vi "duqugongyi.vi"() -> ()   [LabVIEW 2019]
panel:
  in  "树形控件":string(tree)
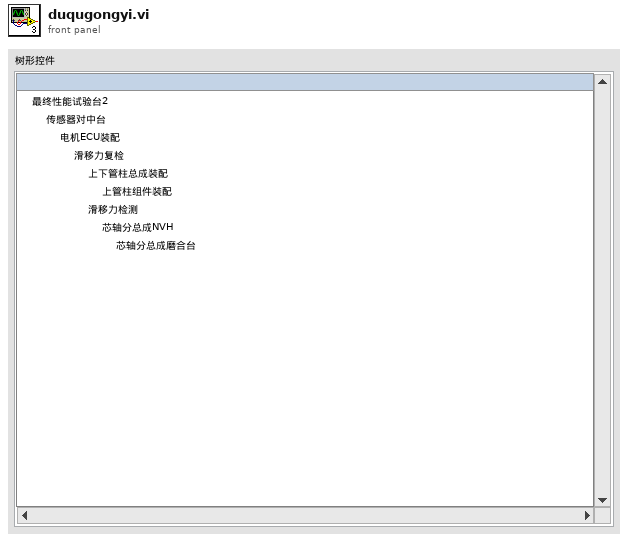
[diagram p1: front panel]
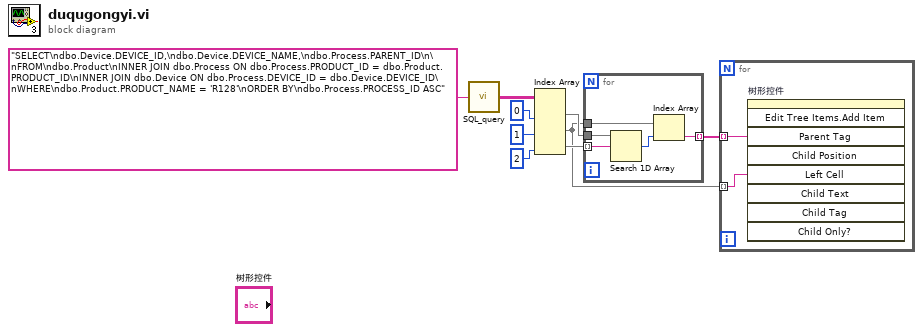
[diagram p0: block diagram]
diagram:
  n1 = call "SQL_query.vi"("SQL query"="SELECT\ndbo.Device.DEVICE_ID,\ndbo.Device.DEVICE_NAME,\ndbo.Process.PARENT_ID\n\nFROM\ndbo.Product\nINNER JOIN dbo.Process ON dbo.Process.PRODUCT_ID = dbo.Product.PRODUCT_ID\nINNER JOIN dbo.Device ON dbo.Process.DEVICE_ID = dbo.Device.DEVICE_ID\nWHERE\ndbo.Product.PRODUCT_NAME = 'R128'\nORDER BY\ndbo.Process.PROCESS_ID ASC") -> ("data"=w8:string[][])  [unwired: 3 in, 1 out]
  n2 = Index Array(array=w8, index (col) #1=0 ("禁用的索引 (列)"), index (col) #2=1 ("索引 (列)"), index (col) #3=2 ("索引 (列)")) -> (element #1=w3:string[], element #2=w1:string[], element #3=w4:string[])  [unwired: 3 in]
  n3 = for {
    tunnel: w1 -> [w12]
    tunnel: w4 -> [w13] mode=indexing
    tunnel: w3 -> [w14]
    tunnel: [w10] -> w2 mode=indexing
    n4 = Search 1D Array(1D array=w14, element=w13) -> (index of element=w11:i32)  [unwired: 1 in]
    n5 = Index Array(array=w12, index=w11) -> (element=w10:string)
  }
  n6 = for {
    tunnel: w2 -> [w15] mode=indexing
    tunnel: w1 -> [w16] mode=indexing
    n7 = invoke on="树形控件" class="Tree (严格)" method="Edit Tree Items.Add Item"("Parent Tag"=w15, "Left Cell"=w16) -> ()  [unwired: 7 in, 9 out]
  }
